vi "rvc Plot Robot.vi"(7 "Reset":bool, 8 "error in (no error)":errorcluster, 10 "joint positions":dbl[](array[numeric]), 11 "NI_Robotics_Serial Robot Arm in":refnum<class "NI_Robotics_Serial Robot Arm.lvclass">) -> (0 "error out":errorcluster, 1 "serial arm out":refnum<class "NI_Robotics_Serial Robot Arm.lvclass">, 2 "forward kinematics":T1, 3 "Scene Object Out":refnum<vi>)   [LabVIEW 2014]
uses:
  <vilib>/Analysis/Matrix/Datatypes/RealMatrix.ctl
  <vilib>/robotics/Kinematics/Robot/NI_Robotics_Serial Robot Arm.lvclass
  <vilib>/robotics/Kinematics/Robot/Forward Kinematics (Point).vi
  <vilib>/picture/3D Picture Control/Object/Create Object (name).vi
  <vilib>/picture/3D Picture Control/Object/Add Object (no reference).vi
  <vilib>/picture/3D Picture Control/Object/Add Object (reference).vi
  <vilib>/robotics/Kinematics/Plotting/NI_Robotics_3DKinematics.lvlib
  <vilib>/picture/3D Picture Control/NI_3D Picture Control.lvlib
  <vilib>/robotics/Kinematics/NI_Kinematics.lvlib
  <vilib>/Analysis/Matrix/NI_Matrix.lvlib
panel:
  out "End Effector transfomation":refnum<vi>
  out "Origin Transformation":refnum<vi>
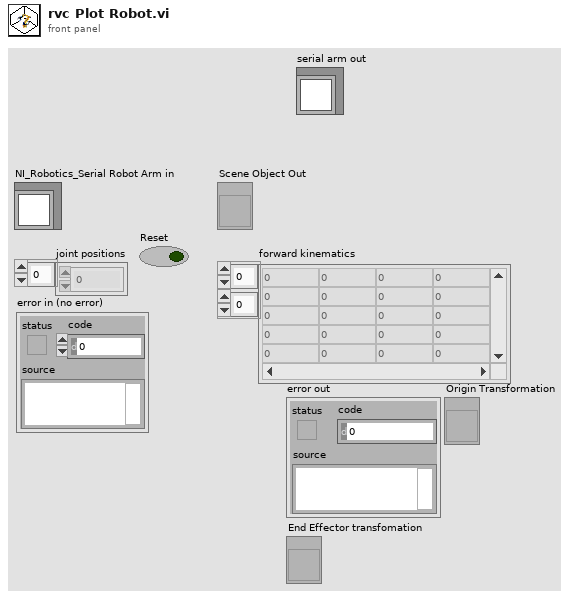
[diagram p1: front panel]
types:
  T1 = typedef "NI_Matrix.lvlib/RealMatrix.ctl" = dbl[][]
  T2 = cluster{"Z Translate":sgl, "Z Translate":sgl, "Z Translate":sgl}
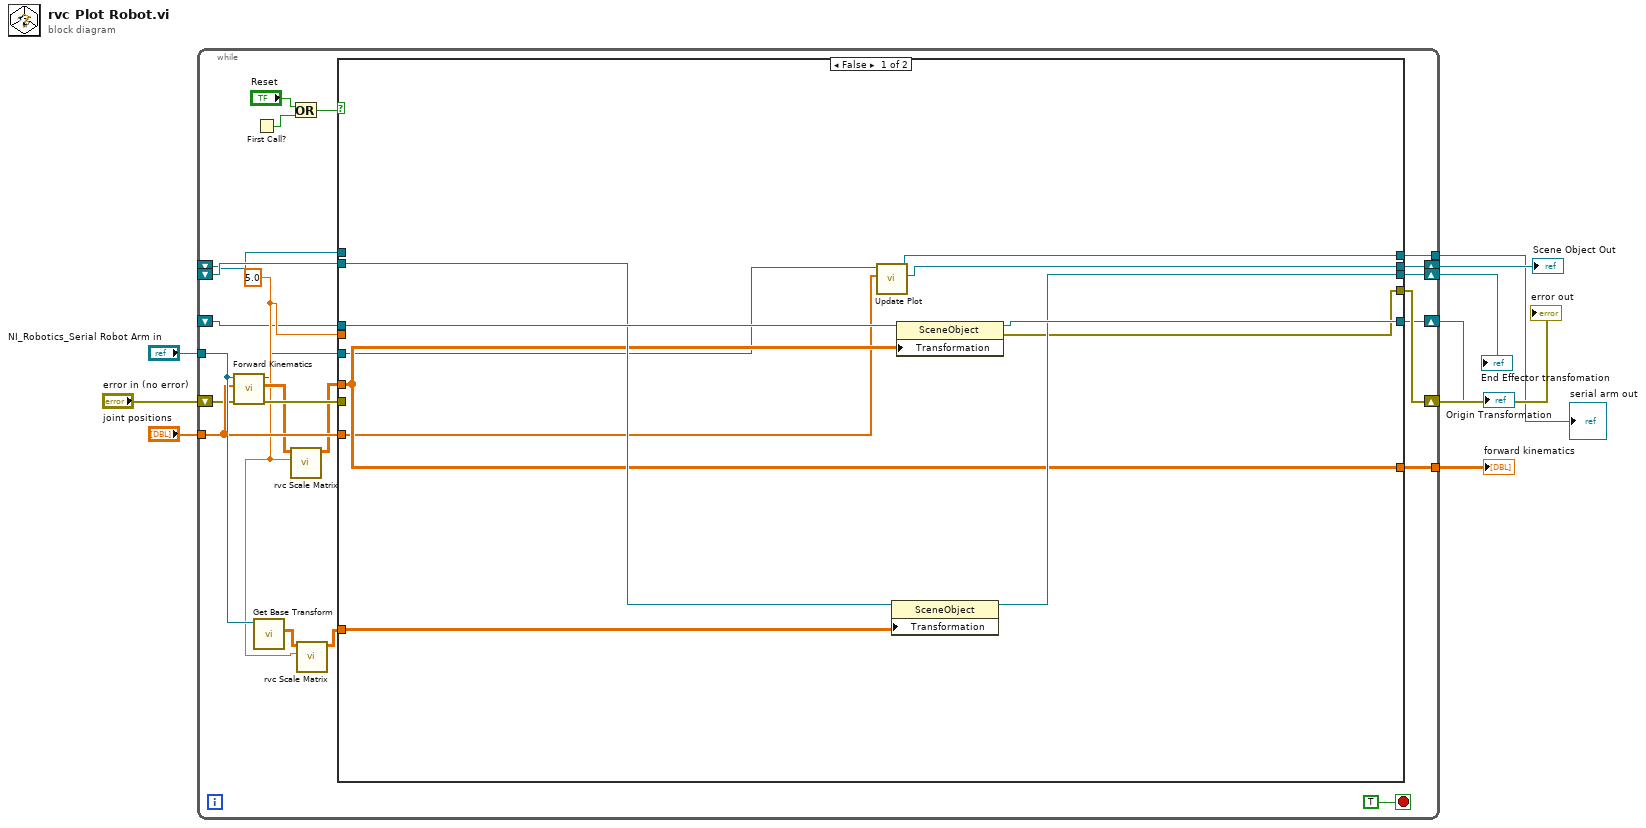
[diagram p0: block diagram]
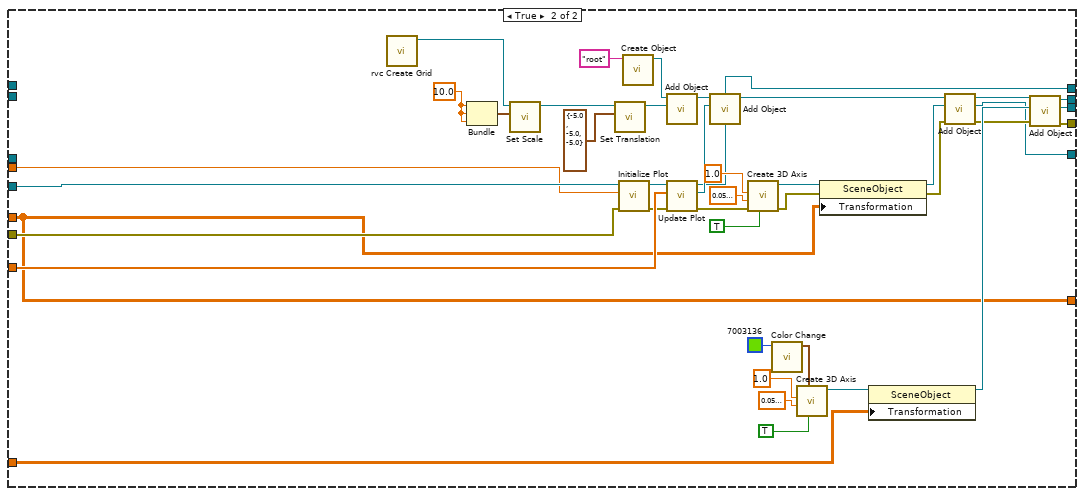
[diagram p2: hidden frame]
diagram:
  n1 = while {
    tunnel: "joint positions" -> [w27]
    tunnel: [w32] -> w8
    tunnel: "NI_Robotics_Serial Robot Arm in" -> [w28]
    shift-right: [w30] -> w5
    shift-left: "error in (no error)" -> [w26]
    shift-right: [w31] -> w6
    shift-left: _ -> [w16]
    shift-right: [w29] -> w2
    shift-left: _ -> [w17]
    shift-right: [w18] -> w3
    shift-left: _ -> [w19]
    tunnel: [w10] -> w1
    stop <- TRUE stop-if-true
    w20 = 5.0 ("scale (1)")
    n2 = call-poly <vilib>:"Forward Kinematics.vi"("error in (no error)"=w26, "joint positions"=w27, "serial arm in"=w28) -> ("error out"=w25:errorcluster, "end effector transform"=w24:T1, "serial arm out"=w11:refnum<class "NI_Robotics_Serial Robot Arm.lvclass">)  [unwired: 6 in]
    n3 = First Call?() -> (First Call?: T/F=w12:bool)
    n4 = call <vilib>:"Get Base Transform.vi"("serial arm in"=w28) -> ("base transform"=w22:T1)  [unwired: 8 in, 2 out]
    n5 = Or(x="Reset", y=w12) -> (x .or. y?=w14:bool)
    n6 = call "rvc Scale Matrix.vi"("scale (1)"=w20, "end effector transform"=w24) -> ("transform"=w23:T1)  [unwired: 9 in]
    n7 = call "rvc Scale Matrix.vi"("scale (1)"=w20, "end effector transform"=w22) -> ("transform"=w21:T1)  [unwired: 9 in]
    n8 = case shown="False" w14 {
      tunnel: w27 -> [w35 w81]
      tunnel: [w37 w48] -> w32
      tunnel: w11 -> [w36 w51]
      tunnel: [w34 w61] -> w31
      tunnel: [w38 w53] -> w30
      tunnel: w25 -> [_ w50]
      tunnel: [w40 w52] -> w29
      tunnel: w23 -> [w37 w48]
      tunnel: w21 -> [w39 w47]
      tunnel: w20 -> [_ w49]
      tunnel: w19 -> [w43 _]
      tunnel: [w42 w46] -> w18
      tunnel: w17 -> [w41 _]
      tunnel: w16 -> [_ _]
      tunnel: [w33 w45] -> w10
      frame False {
        n9 = call <vilib>:"Update Plot.vi"("joint positions"=w35, "serial arm in"=w36) -> ("serial arm scene"=w34:refnum<vi>, "serial arm out"=w33:refnum<class "NI_Robotics_Serial Robot Arm.lvclass">)  [unwired: 7 in, 1 out]
        n10 = property class="SceneObject"(reference=w41, "Transformation"=w39) -> (reference out=w40:refnum<vi>)  [unwired: 1 in, 1 out]
        n11 = property class="SceneObject"(reference=w43, "Transformation"=w37) -> (reference out=w42:refnum<vi>, error out=w38:errorcluster)  [unwired: 1 in]
      }
      frame True {
        w74 = sgl 10.0 ("Z Translate")
        n12 = call "rvc Create Grid.vi"() -> ("SceneObject out"=w75:refnum<vi>)  [unwired: 11 in]
        n13 = Bundle("Z Translate"=w74, "Z Translate"=w74, "Z Translate"=w74) -> (w73:T2)  [unwired: 1 in]
        n14 = call <vilib>:"Set Scale.vi"("Scale"=w73, "Scene Object"=w75) -> ("Scaled Object"=w68:refnum<vi>)  [unwired: 8 in, 1 out]
        n15 = call <vilib>:"Set Translation.vi"("Translation"=cluster{"X":sgl, "Y":sgl, "Z":sgl} {"X"=-5.0, "Y"=-5.0, "Z"=-5.0}, "Scene Object"=w68) -> ("Translated Object"=w67:refnum<vi>)  [unwired: 8 in, 1 out]
        n16 = call <vilib>:"Initialize Plot.vi"("error in (no error)"=w50, "scale (1)"=w49, "serial arm in"=w51) -> ("error out"=w56:errorcluster, "serial arm out"=w76:refnum<class "NI_Robotics_Serial Robot Arm.lvclass">)  [unwired: 7 in]
        n17 = call-poly <vilib>:"Create Object.vi"("Name"="root") -> ("Scene:New Object"=w70:refnum<vi>)  [unwired: 9 in, 1 out]
        n18 = call-poly <vilib>:"Add Object.vi"("New Object In"=w67, "Scene Object In"=w70) -> ("Scene Object Out"=w69:refnum<vi>)  [unwired: 8 in, 1 out]
        n19 = call <vilib>:"Update Plot.vi"("error in (no error)"=w56, "joint positions"=w81, "serial arm in"=w76) -> ("error out"=w79:errorcluster, "serial arm scene"=w72:refnum<vi>, "serial arm out"=w45:refnum<class "NI_Robotics_Serial Robot Arm.lvclass">)  [unwired: 6 in]
        n20 = call-poly <vilib>:"Add Object.vi"("New Object In"=w72, "Scene Object In"=w69) -> ("Scene Object Out"=w44:refnum<vi>)  [unwired: 8 in, 1 out]
        n21 = call <vilib>:"Create 3D Axis.vi"("Axis label?"=TRUE, "error in (no error)"=w79, "Radius"=sgl 0.05, "Length"=sgl 1.0) -> ("error out"=w55:errorcluster, "New Object Refnum"=w83:refnum<vi>)  [unwired: 6 in]
        n22 = call <vilib>:"Color Change.vi"("Color"=u32 7003136) -> ("RGBA"=w58:cluster{"R":sgl, "G":sgl, "B":sgl, "A":sgl})  [unwired: 10 in]
        n23 = call <vilib>:"Create 3D Axis.vi"("Axis label?"=TRUE, "Color"=w58, "Radius"=sgl 0.05, "Length"=sgl 1.0) -> ("New Object Refnum"=w62:refnum<vi>)  [unwired: 6 in, 1 out]
        n24 = property class="SceneObject"(reference=w83, error in=w55, "Transformation"=w48) -> (reference out=w84:refnum<vi>, error out=w80:errorcluster)
        n25 = property class="SceneObject"(reference=w62, "Transformation"=w47) -> (reference out=w59:refnum<vi>)  [unwired: 1 in, 1 out]
        n26 = call-poly <vilib>:"Add Object.vi"("error in (no error)"=w80, "New Object In"=w84, "Scene Object In"=w44) -> ("error out"=w54:errorcluster, "New Object Out"=w46:refnum<vi>, "Scene Object Out"=w60:refnum<vi>)  [unwired: 6 in]
        n27 = call-poly <vilib>:"Add Object.vi"("error in (no error)"=w54, "New Object In"=w59, "Scene Object In"=w60) -> ("error out"=w53:errorcluster, "New Object Out"=w52:refnum<vi>, "Scene Object Out"=w61:refnum<vi>)  [unwired: 6 in]
      }
    }
  }
  "forward kinematics" <- w8
  "Scene Object Out" <- w6
  "error out" <- w5
  "Origin Transformation" <- w3
  "End Effector transfomation" <- w2
  "serial arm out" <- w1
